vi "LWXPS_PositionerSGammaParametersGet.vi"(0 "XPS Reference IN":refnum<k24>, 2 "Positioner Name":string, 5 "LabVIEW error IN":errorcluster) -> (12 "XPS Reference OUT":refnum<k24>, 13 "LabVIEW error OUT":errorcluster, 14 "Returned error code":i32, 15 "Motion velocity":dbl, 16 "Motion acceleration":dbl, 17 "Minimum jerk time":dbl, 18 "Maximum jerk time":dbl, 19 "XPS Error String":string)   [LabVIEW 2014]
uses:
  D:/XPSQ8_LabView_Library/Development/Source/Dll/Newport.XPS.CommandInterface.dll
  Dll/Newport.XPS.CommandInterface.dll
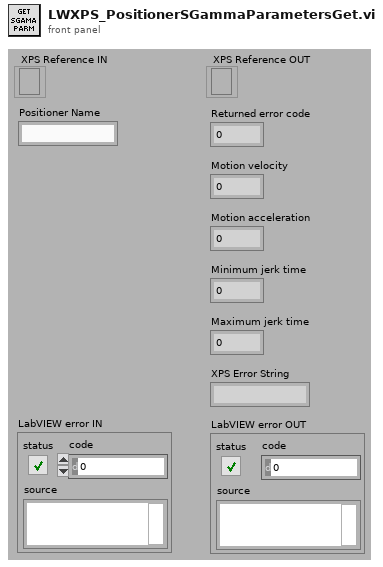
[diagram p1: front panel]
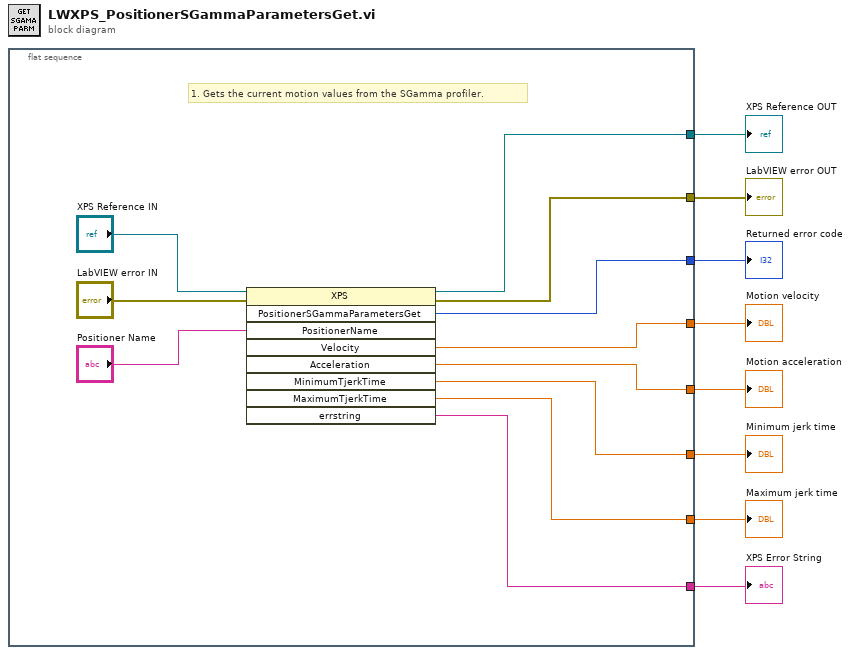
[diagram p0: block diagram]
diagram:
  n1 = flat-sequence {
    tunnel: [w17] -> w8
    tunnel: [w15] -> w7
    tunnel: [w18] -> w6
    tunnel: [w10] -> w3
    tunnel: [w14] -> w5
    tunnel: [w13] -> w2
    tunnel: [w12] -> w1
    tunnel: [w11] -> w4
    frame #0 {
      # "1. Gets the current motion values from the SGamma profiler."
      n2 = invoke class="XPS" method="PositionerSGammaParametersGet"(reference="XPS Reference IN", error in="LabVIEW error IN", "PositionerName"="Positioner Name") -> (reference out=w17:refnum<k24>, error out=w15:errorcluster, "PositionerSGammaParametersGet"=w18:i32, "Velocity"=w10:dbl, "Acceleration"=w14:dbl, "MinimumTjerkTime"=w13:dbl, "MaximumTjerkTime"=w12:dbl, "errstring"=w11:string)  [unwired: 6 in, 1 out]
    }
  }
  "XPS Error String" <- w4
  "XPS Reference OUT" <- w8
  "LabVIEW error OUT" <- w7
  "Returned error code" <- w6
  "Motion acceleration" <- w5
  "Motion velocity" <- w3
  "Minimum jerk time" <- w2
  "Maximum jerk time" <- w1
